vi "Main.vi"() -> ()   [LabVIEW 2015]
doc: "Use this template to build a simple state machine design pattern. Each state executes code and determines which state to transition to."
uses:
  controls/State.ctl
  controls/Data.ctl
panel:
  out "Waveform Chart":dbl[](graph)
  in  "Do Something Else <Replace Me>":bool
  in  "Do Something <Replace Me>":bool caption="Do Something"
  in  "Exit":bool
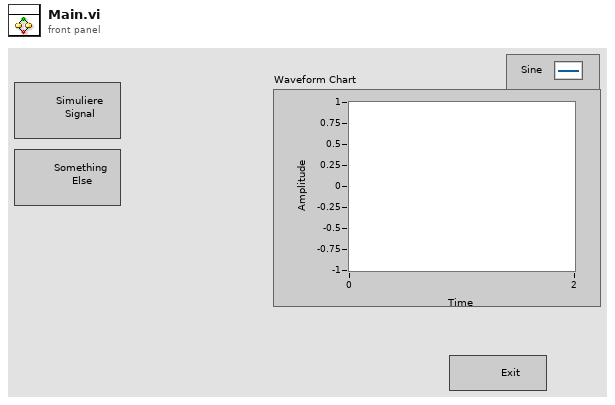
[diagram p1: front panel]
types:
  T1 = typedef "Data.ctl" = cluster{"Boolean ":bool, "String":string, "Signal":dbl[]}
  T2 = typedef "State.ctl" = enum16{"Initialize", "Wait for Event", "Messung Simulieren", "Text verknüpfen", "Exit"}
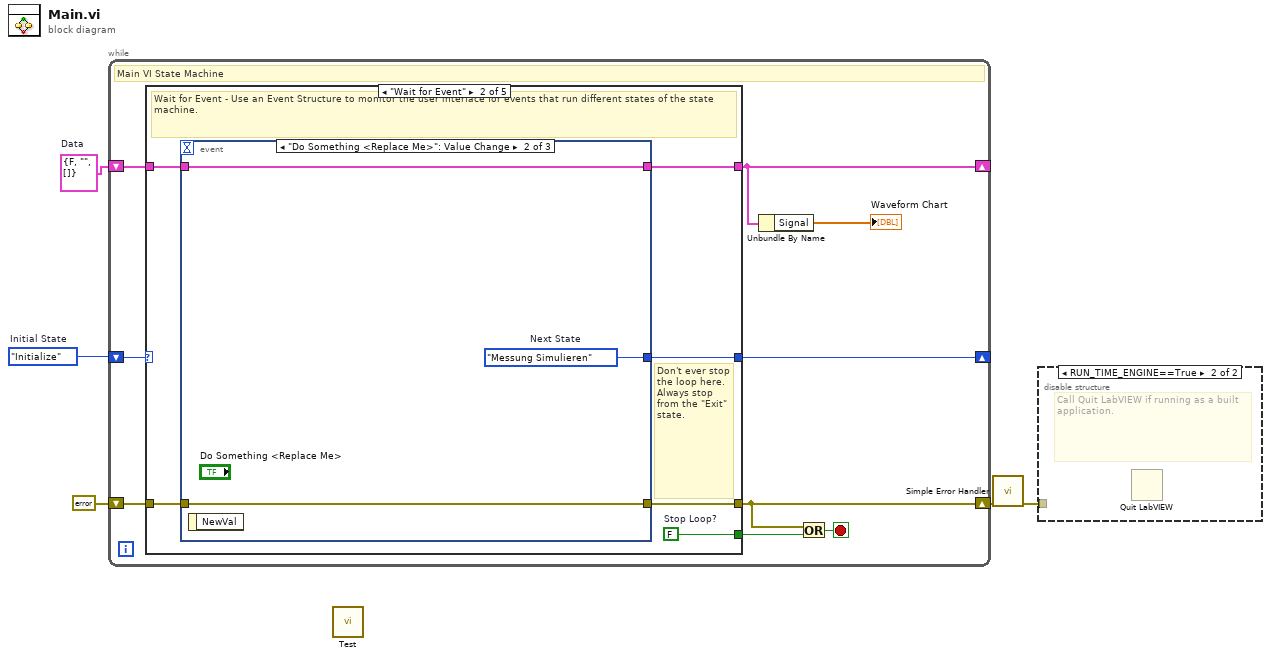
[diagram p0: block diagram]
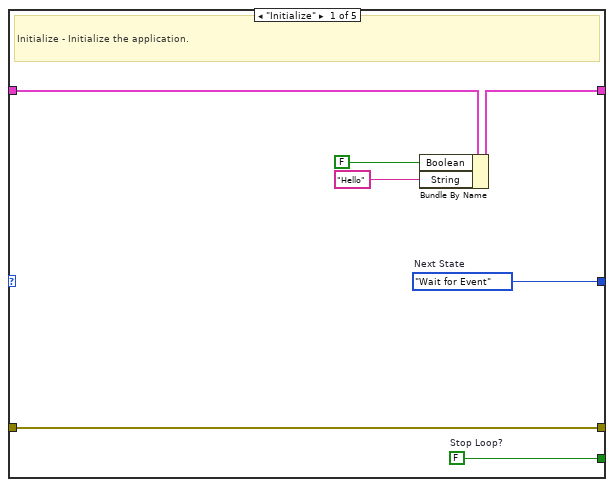
[diagram p3: hidden frame]
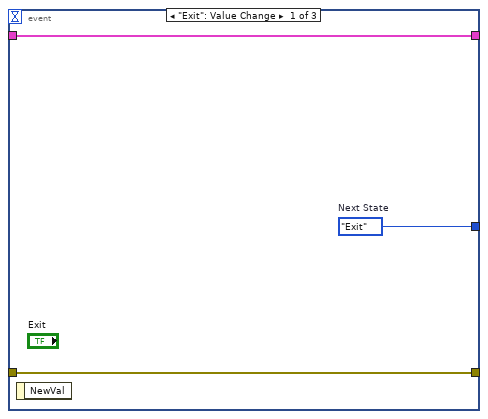
[diagram p4: hidden frame]
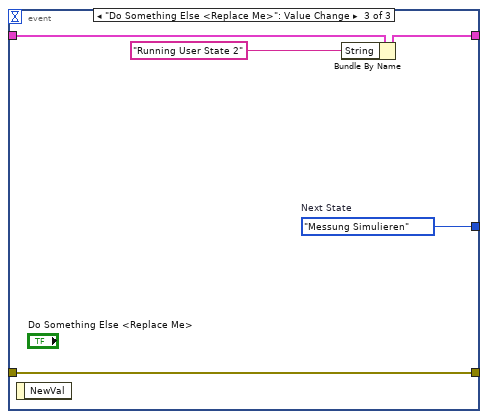
[diagram p5: hidden frame]
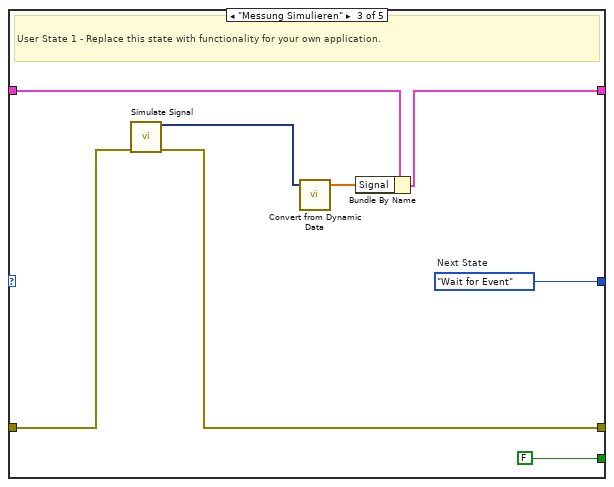
[diagram p6: hidden frame]
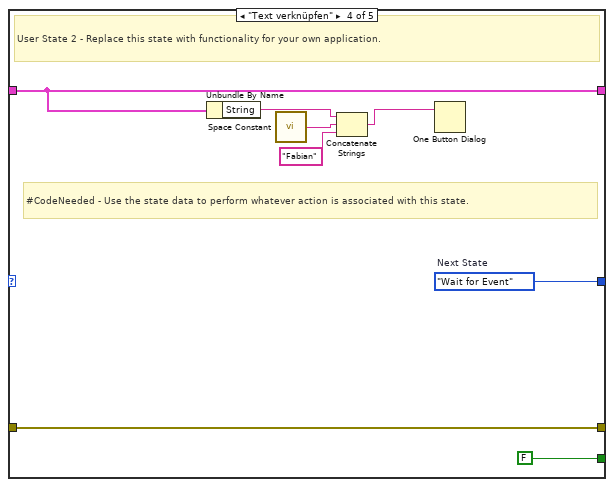
[diagram p7: hidden frame]
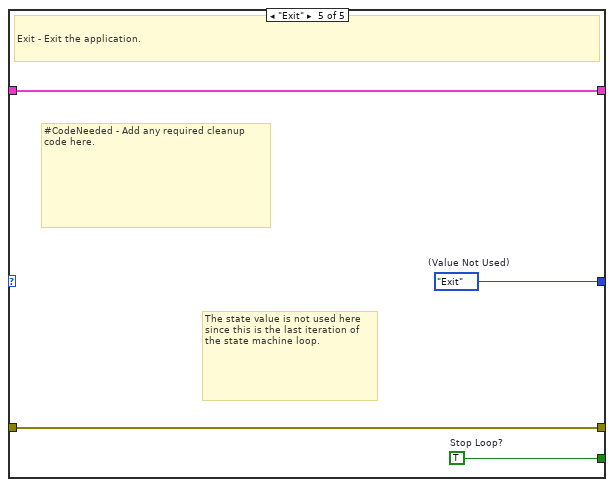
[diagram p8: hidden frame]
diagram:
  w5 = T1 {"Boolean "=FALSE, "String"="", "Signal"=[]}  # Data
  w1 = State."Initialize"  # Initial State
  n1 = while {
    shift-right: [w8] -> _
    shift-left: w1 -> [w9]
    shift-right: [w7] -> _
    shift-left: w5 -> [w14]
    shift-right: [w10] -> w3
    shift-left: errorcluster {"status"=FALSE, "code"=0, "source"=""} ("error constant") -> [w13]
    stop <- w11 stop-if-true
    # "Main VI State Machine"
    n2 = case shown="\"Wait for Event\"" w9 {
      tunnel: [w16 w27 w46 w54 w58] -> w8
      tunnel: [w21 w26 FALSE ("Stop Loop?") FALSE ("Stop Loop?") w56] -> w12
      tunnel: w14 -> [w20 w25 w42 w52 w57]
      tunnel: [w19 w24 w41 w52 w57] -> w7
      tunnel: w13 -> [w17 w23 w40 w51 w55]
      tunnel: [w17 w22 w39 w51 w55] -> w10
      frame "Initialize" {
        w21 = FALSE  # Stop Loop?
        w16 = State."Wait for Event"  # Next State
        # "Initialize - Initialize the application."
        n3 = Bundle By Name(cluster=w20, "Boolean"=FALSE ("Replace_Me_Boolean"), "String"="Hello" ("String <Replace Me>")) -> (w19:T1)
      }
      frame "Wait for Event" {
        w26 = FALSE  # Stop Loop?
        # "Don't ever stop the loop here. Always stop from the \"Exit\" state."
        # "Wait for Event - Use an Event Structure to monitor the user interface for events that run different states of the state machine."
        n4 = event shown="[1] \"Do Something <Replace Me>\": Value Change" {
          selector: _ -> [_ _ _]
          dyn-events: _ -> [_ _ _]
          timeout: _ -> [_ _ _]
          tunnel: [w30 w33 w38] -> w27
          tunnel: w25 -> [w29 w31 w37]
          tunnel: [w29 w31 w36] -> w24
          tunnel: w23 -> [w28 w32 w34]
          tunnel: [w28 w32 w34] -> w22
          event "Exit": Value Change {
            w30 = State."Exit"  # Next State
            n5 = event-data() -> ()  [unwired: 1 in, 1 out]
          }
          event "Do Something <Replace Me>": Value Change {
            w33 = State."Messung Simulieren"  # Next State
            n6 = event-data() -> ()  [unwired: 1 in, 1 out]
          }
          event "Do Something Else <Replace Me>": Value Change {
            w38 = State."Messung Simulieren"  # Next State
            n7 = event-data() -> ()  [unwired: 1 in, 1 out]
            n8 = Bundle By Name(cluster=w37, "String"="Running User State 2" ("Running User State 2")) -> (w36:T1)
          }
        }
      }
      frame "Messung Simulieren" {
        w46 = State."Wait for Event"  # Next State
        # "User State 1 - Replace this state with functionality for your own application."
        n9 = call "Simulate Signal"("error in (no error)"=w40) -> ("Sine"=w44:dynamicdata, "error out"=w39:errorcluster)  [unwired: 13 in]
        n10 = call "Convert from Dynamic Data"("Dynamic Data Type"=w44) -> ("Array"=w43:dbl[])  [unwired: 3 in]
        n11 = Bundle By Name(cluster=w42, "Signal"=w43) -> (w41:T1)
      }
      frame "Text verknüpfen" {
        w54 = State."Wait for Event"  # Next State
        # "#CodeNeeded - Use the state data to perform whatever action is associated with this state."
        # "User State 2 - Replace this state with functionality for your own application."
        n12 = Unbundle By Name(w52) -> ("String"=w50:string)
        n13 = call <vilib>:"Space Constant.vi"() -> ("String"=w49:string)
        n14 = Concatenate Strings(w50, w49, "Fabian" ("string")) -> (w48:string)
        n15 = One Button Dialog(message=w48) -> ()  [unwired: 1 in, 1 out]
      }
      frame "Exit" {
        w56 = TRUE  # Stop Loop?
        w58 = State."Exit"  # (Value Not Used)
        # "#CodeNeeded - Add any required cleanup code here."
        # "The state value is not used here since this is the last iteration of the state machine loop."
        # "Exit - Exit the application."
      }
    }
    n16 = Unbundle By Name(w7) -> ("Signal"=→"Waveform Chart":dbl[])
    n17 = Or(x=w10, y=w12) -> (x .or. y?=w11:bool)
  }
  n18 = call "Test.vi"() -> ()  [unwired: 12 in]
  n19 = call <vilib>:"Simple Error Handler.vi"("error in (no error)"=w3) -> ("error out"=w2:errorcluster)  [unwired: 4 in, 4 out]
  n20 = disable-structure shown="RUN_TIME_ENGINE==True" {
    disable-tunnel: w2 -> [_ _]
    frame condition #0 (active) {
    }
    frame condition #1 {
      # "Call Quit LabVIEW if running as a built application."
      n21 = Quit LabVIEW() -> ()  [unwired: 1 in]
    }
  }
